vi "Get Model Information.vi"(8 "error in":errorcluster, 11 "Alicat Device in":refnum<class "Alicat Device.lvclass">) -> (0 "error out":errorcluster, 2 "DataOut":string, 3 "Alicat Device out":refnum<class "Alicat Device.lvclass">)   [LabVIEW 2019, in "Alicat Device.lvclass"]
doc: "Retrieve the model data from the Alicat device using the command <b>X??M*</b> where <b>X</b> is the address of the device. The model data will contain all the information to determine what the device is. This includes the scale, units and model."
uses:
  Alicat Device.lvclass
  Reusable/Session APIs/Serial/Serial Session.lvclass
  C:/Program Files (x86)/National Instruments/LabVIEW 2019/vi.lib/MSR Consulting, LLC/General Reuse/Session APIs/_Session Fwk/Session - Root.lvclass
  Alicat Device.lvclass/Alicat Device.ctl
  Reusable/Session APIs/Serial/Public/Get Multiline Str.vi
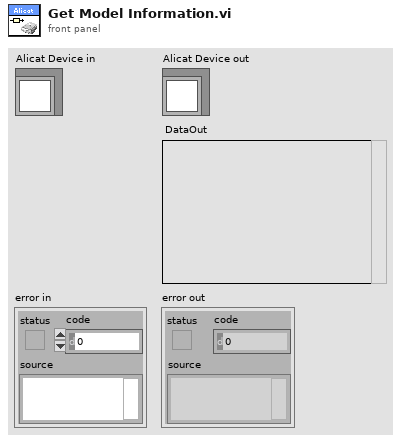
[diagram p1: front panel]
types:
  T1 = typedef "Session - Root.lvclass/Session Handle.ctl" = refnum<data-value>
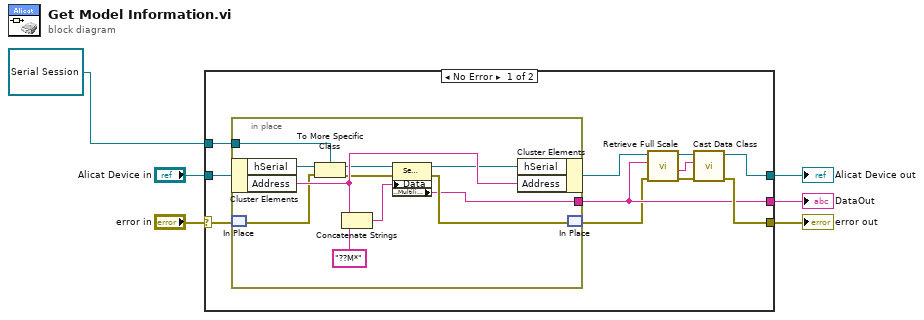
[diagram p0: block diagram]
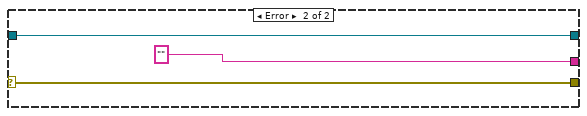
[diagram p2: hidden frame]
diagram:
  n1 = case shown="No Error" "error in" {
    selector: "error in" -> [w16 w31]
    tunnel: "Alicat Device in" -> [w17 w30]
    tunnel: [w15 w31] -> w3
    tunnel: [w14 w30] -> w5
    tunnel: [w13 "" ("DataOut")] -> w2
    tunnel: refnum<data-value> refnum ("hSerial") -> [w11 _]
    frame No Error {
      n2 = in-place {
        in-place-border: [w23] -> w13
        in-place-border: w11 -> [w21]
        n3 = in-place-cluster #1(w17) -> ("hSerial"=w22:T1, "Address"=w28:string)
        n4 = in-place-match #2(w16) -> (w19:errorcluster)
        n5 = To More Specific Class(target class=w21, reference=w22, error in=w19) -> (specific class reference=w20:refnum<data-value>, error out=w18:errorcluster)
        n6 = Concatenate Strings(w28, "??M*" ("string")) -> (w26:string)
        n7 = property class="Serial Session"(reference=w20, error in=w18, "Data"=w26) -> (reference out=w25:refnum<data-value>, error out=w24:errorcluster, "Public:Multiline Str"=w23:string)
        n8 = in-place-cluster #1("hSerial"=w25, "Address"=w28) -> (w12:refnum<class "Alicat Device.lvclass">)
        n9 = in-place-match #2(w24) -> (w7:errorcluster)
      }
      n10 = call "Retrieve Full Scale.vi"("error in"=w7, "Model Data"=w13, "Alicat Device in"=w12) -> ("error out"=w9:errorcluster, "Type"=w8:string, "Alicat Device out"=w10:refnum<class "Alicat Device.lvclass">)  [unwired: 5 in, 1 out]
      n11 = call "Cast Data Class.vi"("error in"=w9, "Type"=w8, "Alicat Device in"=w10) -> ("error out"=w15:errorcluster, "Alicat Device out"=w14:refnum<class "Alicat Device.lvclass">)  [unwired: 6 in, 1 out]
    }
    frame Error {
    }
  }
  "error out" <- w3
  "Alicat Device out" <- w5
  "DataOut" <- w2
